vi "if_l0.vi"() -> ()   [LabVIEW 2009]
uses:
  <vilib>/Platform/portaccess.llb/Out Port8.vi
panel:
  out "Array":bool[](array[boolean])=[FALSE, FALSE, TRUE, TRUE, FALSE, TRUE, TRUE, TRUE]
  in  "Numeric 4":u8=127
  in  "Numeric 3":u8=55
  in  "Numeric 2":u8=147
  in  "Numeric":u8=78
  in  "Boolean 2":bool
  in  "Boolean":bool=TRUE
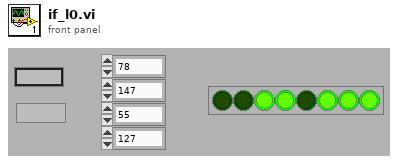
[diagram p1: front panel]
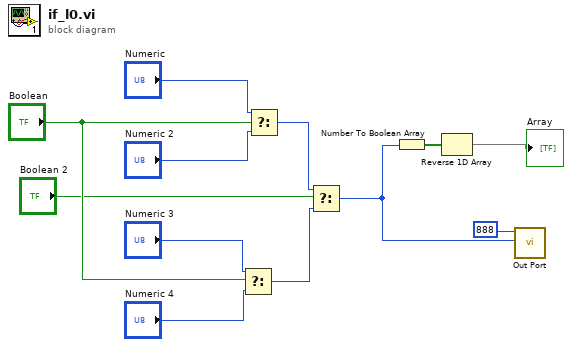
[diagram p0: block diagram]
diagram:
  n1 = Select(t="Numeric 3", s="Boolean", f="Numeric 4") -> (s? t:f=w3:u8)
  n2 = Select(t="Numeric", s="Boolean", f="Numeric 2") -> (s? t:f=w4:u8)
  n3 = Select(t=w4, s="Boolean 2", f=w3) -> (s? t:f=w1:u8)
  n4 = Number To Boolean Array(number=w1) -> (Boolean array=w12:bool[])
  n5 = Reverse 1D Array(array=w12) -> (reversed array=→"Array":bool[])
  n6 = call-poly <vilib>:"Out Port.vi"("write value"=w1, "address"=888) -> ()  [unwired: 7 in, 1 out]
